vi "Extract Fiducial Definitions.vi"(8 "error in":errorcluster, 10 "Part Name":string, 11 "Config Location":path) -> (0 "error out":errorcluster, 2 "Feature Definitions":T1(array[cluster]))   [LabVIEW 2011]
uses:
  Vec3d Class/Vec3d Class.lvclass
  <vilib>/Utility/config.llb/Read Key (String).vi
  <vilib>/Utility/config.llb/NI_LVConfig.lvlib
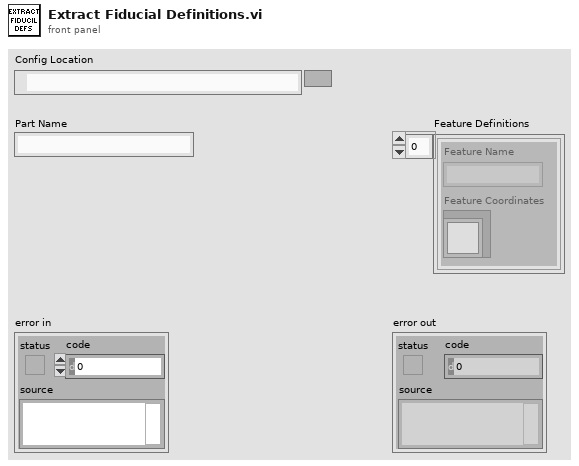
[diagram p1: front panel]
types:
  T1 = cluster{"Feature Coordinates":refnum<class "Vec3d Class.lvclass">, "Feature Name":string}[]
  T2 = typedef "NI_LVConfig.lvlib/Config Data RefNum.ctl" = refnum<k1>
  T3 = cluster{"Feature Coordinates":refnum<class "Vec3d Class.lvclass">, "Feature Name":string}
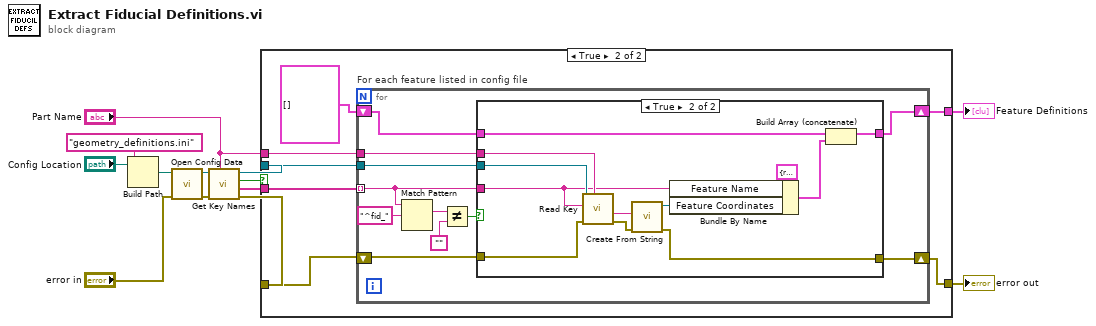
[diagram p0: block diagram]
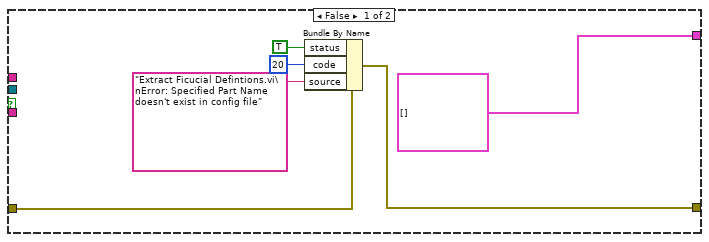
[diagram p2: hidden frame]
diagram:
  n1 = Build Path(base path="Config Location", name or relative path="geometry_definitions.ini") -> (appended path=w12:path)
  n2 = call <vilib>:"Open Config Data.vi"("error in (no error)"="error in", "configuration file path"=w12) -> ("error out"=w8:errorcluster, "refnum"=w9:T2)  [unwired: 7 in, 1 out]
  n3 = call <vilib>:"Get Key Names.vi"("section"="Part Name", "error in (no error)"=w8, "refnum"=w9) -> ("error out"=w6:errorcluster, "key names"=w4:string[], "section exists?"=w7:bool, "refnum out"=w3:T2)  [unwired: 5 in]
  n4 = case shown="True" w7 {
    tunnel: w6 -> [w19 w23]
    tunnel: [w15 w22] -> w5
    tunnel: w4 -> [_ w25]
    tunnel: w3 -> [_ w26]
    tunnel: "Part Name" -> [_ w24]
    tunnel: [T1 [] w21] -> w1
    frame False {
      n5 = Bundle By Name(cluster=w19, "status"=TRUE, "code"=20, "source"="Extract Ficucial Defintions.vi\nError: Specified Part Name doesn't exist in config file") -> (w15:errorcluster)
    }
    frame True {
      n6 = for "For each feature listed in config file" {
        tunnel: w26 -> [w37]
        tunnel: w25 -> [w33] mode=indexing
        tunnel: w24 -> [w36]
        shift-right: [w34] -> w22
        shift-left: w23 -> [w35]
        shift-right: [w27] -> w21
        shift-left: T1 [] -> [w28]
        n7 = Match Pattern(string=w33, regular expression="^fid_") -> (match substring=w31:string)  [unwired: 1 in, 3 out]
        n8 = Not Equal?(x=w31, y="") -> (x != y?=w29:bool)
        n9 = case shown="True" w29 {
          tunnel: w37 -> [_ w51]
          tunnel: w36 -> [_ w50]
          tunnel: w35 -> [w38 w47]
          tunnel: [w38 w44] -> w34
          tunnel: w33 -> [_ w43]
          tunnel: w28 -> [w39 w42]
          tunnel: [w39 w40] -> w27
          frame False {
          }
          frame True {
            n10 = call-poly <vilib>:"Read Key.vi"("section"=w50, "error in (no error)"=w47, "key"=w43, "refnum"=w51) -> ("error out"=w48:errorcluster, "value"=w49:string)  [unwired: 4 in, 2 out]
            n11 = call "Create From String.vi"("error in"=w48, "Input String"=w49) -> ("error out"=w44:errorcluster, "Vec3d out"=w45:refnum<class "Vec3d Class.lvclass">)  [unwired: 8 in]
            n12 = Bundle By Name(cluster=T3 {"Feature Coordinates"=refnum, "Feature Name"=""} ("Feature Description"), "Feature Name"=w43, "Feature Coordinates"=w45) -> (w41:T3)
            n13 = Build Array (concatenate)(w42, w41) -> (w40:T1)
          }
        }
      }
    }
  }
  "Feature Definitions" <- w1
  "error out" <- w5
